vi "Read displacements.vi"(8 "error in (no error)":errorcluster, 11 "MotorSim in":refnum<class "MotorSim.lvclass">) -> (0 "error out":errorcluster, 2 "displacements":T1(array[cluster]), 3 "MotorSim out":refnum<class "MotorSim.lvclass">)   [LabVIEW 2018, in "MotorSim.lvclass"]
uses:
  MotorSim.lvclass
  MotorSim.lvclass/MotorSim.ctl
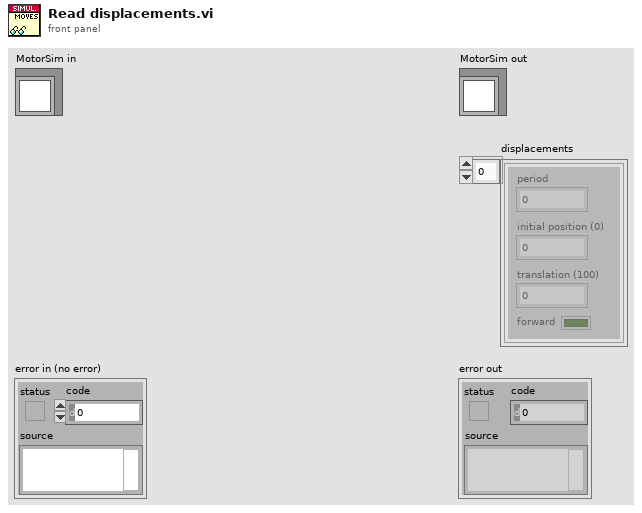
[diagram p1: front panel]
types:
  T1 = cluster{"period":u32, "initial position (0)":i32, "translation (100)":i32, "forward":bool}[]
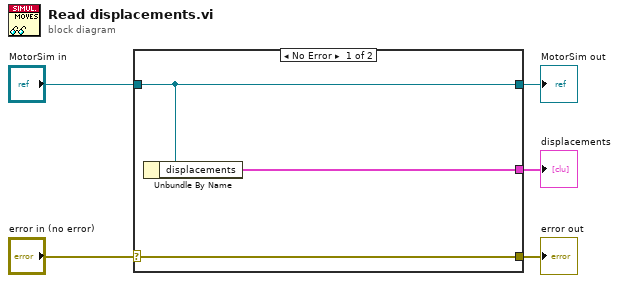
[diagram p0: block diagram]
diagram:
  n1 = case shown="No Error" "error in (no error)" {
    selector: "error in (no error)" -> [w8 w9]
    tunnel: [w8 w9] -> w4
    tunnel: [w7 w10] -> w2
    tunnel: "MotorSim in" -> [w7 w10]
    tunnel: [w6 _] -> w1
    frame No Error {
      n2 = Unbundle By Name(w7) -> ("displacements"=w6:T1)
    }
    frame Error {
    }
  }
  "error out" <- w4
  "MotorSim out" <- w2
  "displacements" <- w1
